vi "libssh2_sftp_init.vi"(8 "error in (no error)":errorcluster, 11 "session":T2) -> (0 "error out":errorcluster, 3 "sftp":T1)   [LabVIEW 2013, in "libssh2.lvlib"]
doc: "Initialize an SFTP session."
uses:
  libssh2.lvlib
  Session Refnum.ctl
  SFTP Refnum.ctl
  Not A Session.vi
  <vilib>/Utility/error.llb/Error Cluster From Error Code.vi
  Global Settings.vi
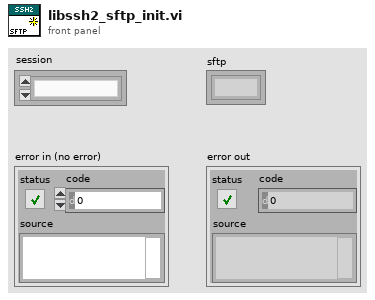
[diagram p1: front panel]
types:
  T1 = typedef "libssh2.lvlib/SFTP Refnum.ctl" = refnum<k1>
  T2 = typedef "libssh2.lvlib/Session Refnum.ctl" = refnum<k1>
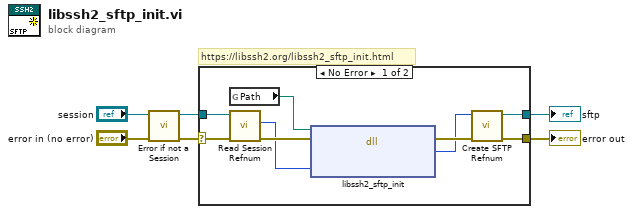
[diagram p0: block diagram]
diagram:
  # "https://libssh2.org/libssh2_sftp_init.html"
  n1 = call "Error if not a Session.vi"("error in (no error)"="error in (no error)", "session"="session") -> ("error out"=w4:errorcluster, "session out"=w3:T2)  [unwired: 8 in]
  n2 = case shown="No Error" w4 {
    selector: w4 -> [w14 w16]
    tunnel: w3 -> [w13 _]
    tunnel: [w9 w16] -> w2
    tunnel: [w7 _] -> w1
    frame No Error {
      n3 = global read "Global Settings.vi" "Path"() -> (w15:path)
      n4 = call "Read Session Refnum.vi"("error in (no error)"=w14, "session"=w13) -> ("error out"=w12:errorcluster, "LIBSSH2_SESSION*"=w11:u64)  [unwired: 5 in, 3 out]
      n5 = dll-call lib="?" fn="libssh2_sftp_init"(path in=w15, error in=w12, "session"=w11) -> (error out=w10:errorcluster, "return value"=w8:u64)  [unwired: 2 in, 1 out]
      n6 = call "Create SFTP Refnum.vi"("error in (no error)"=w10, "LIBSSH2_SFTP*"=w8) -> ("error out"=w9:errorcluster, "sftp"=w7:T1)  [unwired: 8 in]
    }
    frame Error {
    }
  }
  "error out" <- w2
  "sftp" <- w1
